vi "计时.vi"(11 "初始化？":bool) -> (2 "时间计数(S)":dbl, 3 "启动时间":dbl)   [LabVIEW 2020]
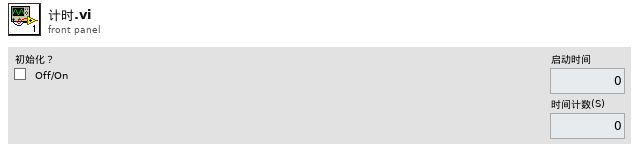
[diagram p1: front panel]
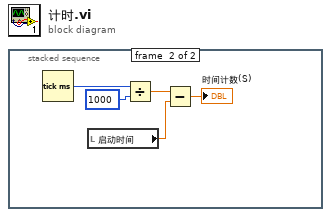
[diagram p0: block diagram]
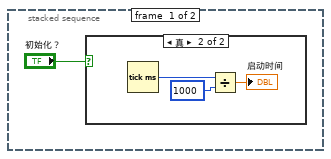
[diagram p2: hidden frame]
diagram:
  n1 = stacked-sequence {
    frame #0 {
      n2 = case shown="真" "初始化？" {
        frame False {
        }
        frame True {
          n3 = Tick Count (ms)() -> (millisecond timer value=w4:u32)
          n4 = Divide(x=w4, y=u32 1000) -> (x/y=→"启动时间":dbl)
        }
      }
    }
    frame #1 {
      n5 = Tick Count (ms)() -> (millisecond timer value=w9:u32)
      n6 = local read "启动时间"() -> (w6:dbl)
      n7 = Divide(x=w9, y=u32 1000) -> (x/y=w5:dbl)
      n8 = Subtract(x=w5, y=w6) -> (x-y=→"时间计数(S)":dbl)
    }
  }
